vi "ButtonPress.vi"(1 "Button":bool) -> (0 "JustPressed":bool)   [LabVIEW 2014]
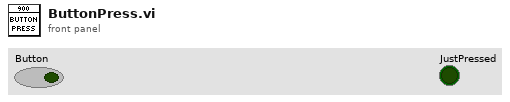
[diagram p1: front panel]
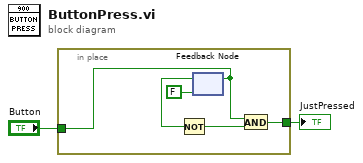
[diagram p0: block diagram]
diagram:
  n1 = in-place {
    in-place-border: [w4] -> w1
    in-place-border: "Button" -> [w3]
    n2 = feedback #1(FALSE ("B")) -> (w6:bool)
    n3 = Not(x=w6) -> (.not. x?=w5:bool)
    n4 = feedback-in #1(w3) -> ()
    n5 = And(x=w3, y=w5) -> (x .and. y?=w4:bool)
  }
  "JustPressed" <- w1
